vi "read tag bus from cvt.vi"(9 "Indices":i32[](array[numeric]), 10 "Data Type":T1, 11 "data table in":T2) -> (3 "data table out":T2)   [LabVIEW 2013, in "TEC runtime.lvclass"]
uses:
  TEC runtime.lvclass
  <vilib>/NI/Tag Bus/table/data table.ctl
  <vilib>/NI/Current Value Table/Type Defs/Data Types.ctl
  <vilib>/NI/Current Value Table/DataTypes/Double_Read Index Set.vi
  <vilib>/NI/Current Value Table/DataTypes/Array of String_Read Index Set.vi
  <vilib>/NI/Current Value Table/DataTypes/Array of Boolean_Read Index Set.vi
  <vilib>/NI/Current Value Table/DataTypes/Array of Single_Read Index Set.vi
  <vilib>/NI/Current Value Table/DataTypes/Array of Double_Read Index Set.vi
  <vilib>/NI/Current Value Table/DataTypes/Array of I8_Read Index Set.vi
  <vilib>/NI/Current Value Table/DataTypes/Array of I16_Read Index Set.vi
  <vilib>/NI/Current Value Table/DataTypes/Array of I32_Read Index Set.vi
  <vilib>/NI/Current Value Table/DataTypes/Array of I64_Read Index Set.vi
  <vilib>/NI/Current Value Table/DataTypes/Array of U64_Read Index Set.vi
  <vilib>/NI/Current Value Table/DataTypes/Array of U32_Read Index Set.vi
  <vilib>/NI/Current Value Table/DataTypes/Array of U16_Read Index Set.vi
  <vilib>/NI/Current Value Table/DataTypes/Array of U8_Read Index Set.vi
  <vilib>/NI/Current Value Table/DataTypes/Boolean_Read Index Set.vi
  <vilib>/NI/Current Value Table/DataTypes/String_Read Index Set.vi
  <vilib>/NI/Current Value Table/DataTypes/U8_Read Index Set.vi
  <vilib>/NI/Current Value Table/DataTypes/U16_Read Index Set.vi
  <vilib>/NI/Current Value Table/DataTypes/U32_Read Index Set.vi
  <vilib>/NI/Current Value Table/DataTypes/U64_Read Index Set.vi
  <vilib>/NI/Current Value Table/DataTypes/I8_Read Index Set.vi
  <vilib>/NI/Current Value Table/DataTypes/I16_Read Index Set.vi
  <vilib>/NI/Current Value Table/DataTypes/I32_Read Index Set.vi
  <vilib>/NI/Current Value Table/DataTypes/I64_Read Index Set.vi
  <vilib>/NI/Current Value Table/DataTypes/Single_Read Index Set.vi
  <vilib>/NI/Current Value Table/Memory Block.vi
  <vilib>/NI/Current Value Table/DataTypes/Double_Memory Block.vi
  <vilib>/NI/Current Value Table/DataTypes/Array of String_Memory Block.vi
  <vilib>/NI/Current Value Table/DataTypes/Array of Boolean_Memory Block.vi
  <vilib>/NI/Current Value Table/DataTypes/Array of Single_Memory Block.vi
  <vilib>/NI/Current Value Table/DataTypes/Array of Double_Memory Block.vi
  <vilib>/NI/Current Value Table/DataTypes/Array of I8_Memory Block.vi
  <vilib>/NI/Current Value Table/DataTypes/Array of I16_Memory Block.vi
  <vilib>/NI/Current Value Table/DataTypes/Array of I32_Memory Block.vi
  <vilib>/NI/Current Value Table/DataTypes/Array of I64_Memory Block.vi
  <vilib>/NI/Current Value Table/DataTypes/Array of U64_Memory Block.vi
  <vilib>/NI/Current Value Table/DataTypes/Array of U32_Memory Block.vi
  <vilib>/NI/Current Value Table/DataTypes/Array of U16_Memory Block.vi
  <vilib>/NI/Current Value Table/DataTypes/Array of U8_Memory Block.vi
  <vilib>/NI/Current Value Table/DataTypes/Boolean_Memory Block.vi
  <vilib>/NI/Current Value Table/DataTypes/String_Memory Block.vi
  <vilib>/NI/Current Value Table/DataTypes/U8_Memory Block.vi
  <vilib>/NI/Current Value Table/DataTypes/U16_Memory Block.vi
  <vilib>/NI/Current Value Table/DataTypes/U32_Memory Block.vi
  <vilib>/NI/Current Value Table/DataTypes/U64_Memory Block.vi
  <vilib>/NI/Current Value Table/DataTypes/I8_Memory Block.vi
  <vilib>/NI/Current Value Table/DataTypes/I16_Memory Block.vi
  <vilib>/NI/Current Value Table/DataTypes/I32_Memory Block.vi
  <vilib>/NI/Current Value Table/DataTypes/I64_Memory Block.vi
  <vilib>/NI/Current Value Table/DataTypes/Single_Memory Block.vi
  <vilib>/NI/Current Value Table/Current Value Table.lvlib
  <vilib>/NI/Tag Bus/table/data table.lvlib
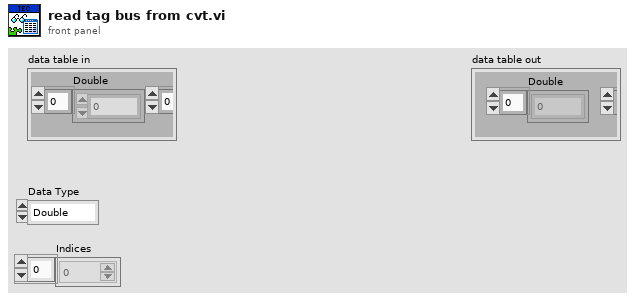
[diagram p1: front panel]
types:
  T1 = typedef "Current Value Table.lvlib/Data Types.ctl" = enum16{"Double", "Single", "I64", "I32", "I16", "I8", "U64", "U32", "U16", "U8", "String", "Boolean", "Array of U8", "Array of U16", "Array of U32", "Array of U64", "Array of I64", "Array of I32", "Array of I16", "Array of I8", "Array of Double", "Array of Single", "Array of Boolean", "Array of String"}
  T2 = typedef "tag bus.lvlib/data table.lvlib/data table.ctl" = cluster{"Double":dbl[], "Single":sgl[], "I64":i64[], "I32":i32[], "I16":i16[], "I8":i8[], "U64":u64[], "U32":u32[], "U16":u16[], "U8":u8[], "Boolean":bool[], "String":string[], "Array of Double":cluster{"DBL Array":dbl[]}[], "Array of Single":cluster{"SGL Array":sgl[]}[], "Array of I64":cluster{"I64 Array":i64[]}[], "Array of I32":cluster{"I32 Array":i32[]}[], "Array of I16":cluster{"I16 Array":i16[]}[], "Array of I8":cluster{"I8 Array":i8[]}[], "Array of U64":cluster{"U64 Array":u64[]}[], "Array of U32":cluster{"U32 Array":u32[]}[], "Array of U16":cluster{"U16 Array":u16[]}[], "Array of U8":cluster{"U8 Array":u8[]}[], "Array of Boolean":cluster{"Boolean Array":bool[]}[], "Array of String":cluster{"String Array":string[]}[]}
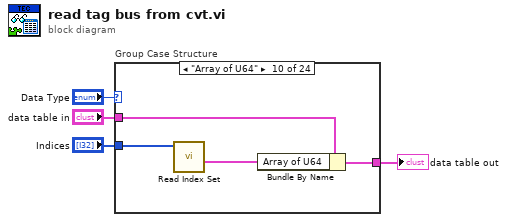
[diagram p0: block diagram]
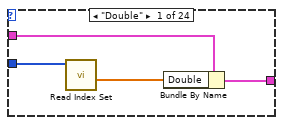
[diagram p2: hidden frame]
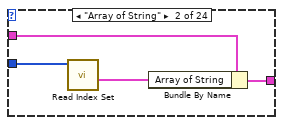
[diagram p3: hidden frame]
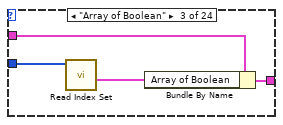
[diagram p4: hidden frame]
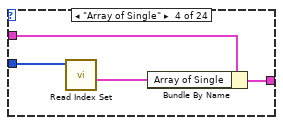
[diagram p5: hidden frame]
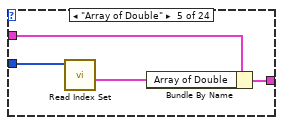
[diagram p6: hidden frame]
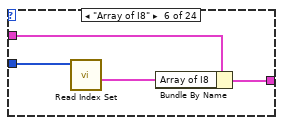
[diagram p7: hidden frame]
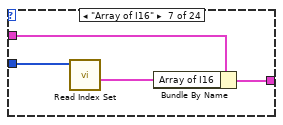
[diagram p8: hidden frame]
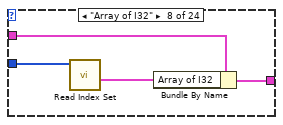
[diagram p9: hidden frame]
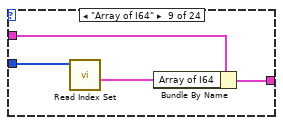
[diagram p10: hidden frame]
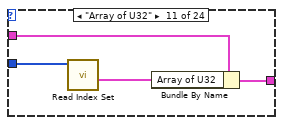
[diagram p11: hidden frame]
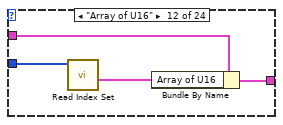
[diagram p12: hidden frame]
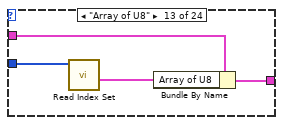
[diagram p13: hidden frame]
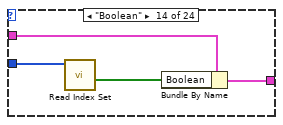
[diagram p14: hidden frame]
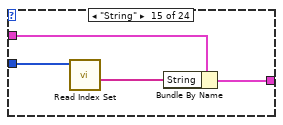
[diagram p15: hidden frame]
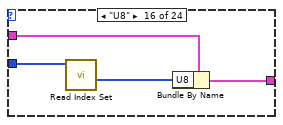
[diagram p16: hidden frame]
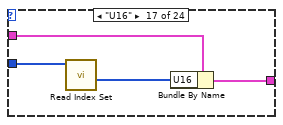
[diagram p17: hidden frame]
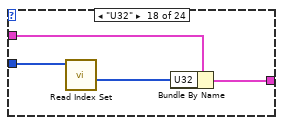
[diagram p18: hidden frame]
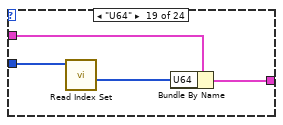
[diagram p19: hidden frame]
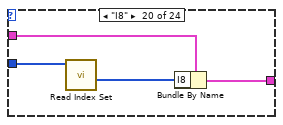
[diagram p20: hidden frame]
diagram:
  n1 = case "Group Case Structure" shown="\"Array of U64\"" "Data Type" {
    tunnel: "Indices" -> [w8 w12 w16 w20 w24 w28 w32 w36 w40 w44 w48 w52 w56 w60 w64 w68 w72 w76 w80 w84 w88 w92 w96 w100]
    tunnel: "data table in" -> [w7 w11 w15 w19 w23 w27 w31 w35 w39 w43 w47 w51 w55 w59 w63 w67 w71 w75 w79 w83 w87 w91 w95 w99]
    tunnel: [w6 w10 w14 w18 w22 w26 w30 w34 w38 w42 w46 w50 w54 w58 w62 w66 w70 w74 w78 w82 w86 w90 w94 w98] -> w3
    frame "Double" {
      n2 = call-poly <vilib>:"Read Index Set.vi"("Indices"=w8) -> ("Values"=w5:dbl[])  [unwired: 10 in]
      n3 = Bundle By Name(cluster=w7, "Double"=w5) -> (w6:T2)
    }
    frame "Array of String" {
      n4 = call-poly <vilib>:"Read Index Set.vi"("Indices"=w12) -> ("Values"=w9:cluster{"String Array":string[]}[])  [unwired: 10 in]
      n5 = Bundle By Name(cluster=w11, "Array of String"=w9) -> (w10:T2)
    }
    frame "Array of Boolean" {
      n6 = call-poly <vilib>:"Read Index Set.vi"("Indices"=w16) -> ("Values"=w13:cluster{"Boolean Array":bool[]}[])  [unwired: 10 in]
      n7 = Bundle By Name(cluster=w15, "Array of Boolean"=w13) -> (w14:T2)
    }
    frame "Array of Single" {
      n8 = call-poly <vilib>:"Read Index Set.vi"("Indices"=w20) -> ("Values"=w17:cluster{"SGL Array":sgl[]}[])  [unwired: 10 in]
      n9 = Bundle By Name(cluster=w19, "Array of Single"=w17) -> (w18:T2)
    }
    frame "Array of Double" {
      n10 = call-poly <vilib>:"Read Index Set.vi"("Indices"=w24) -> ("Values"=w21:cluster{"DBL Array":dbl[]}[])  [unwired: 10 in]
      n11 = Bundle By Name(cluster=w23, "Array of Double"=w21) -> (w22:T2)
    }
    frame "Array of I8" {
      n12 = call-poly <vilib>:"Read Index Set.vi"("Indices"=w28) -> ("Values"=w25:cluster{"I8 Array":i8[]}[])  [unwired: 10 in]
      n13 = Bundle By Name(cluster=w27, "Array of I8"=w25) -> (w26:T2)
    }
    frame "Array of I16" {
      n14 = call-poly <vilib>:"Read Index Set.vi"("Indices"=w32) -> ("Values"=w29:cluster{"I16 Array":i16[]}[])  [unwired: 10 in]
      n15 = Bundle By Name(cluster=w31, "Array of I16"=w29) -> (w30:T2)
    }
    frame "Array of I32" {
      n16 = call-poly <vilib>:"Read Index Set.vi"("Indices"=w36) -> ("Values"=w33:cluster{"I32 Array":i32[]}[])  [unwired: 10 in]
      n17 = Bundle By Name(cluster=w35, "Array of I32"=w33) -> (w34:T2)
    }
    frame "Array of I64" {
      n18 = call-poly <vilib>:"Read Index Set.vi"("Indices"=w40) -> ("Values"=w37:cluster{"I64 Array":i64[]}[])  [unwired: 10 in]
      n19 = Bundle By Name(cluster=w39, "Array of I64"=w37) -> (w38:T2)
    }
    frame "Array of U64" {
      n20 = call-poly <vilib>:"Read Index Set.vi"("Indices"=w44) -> ("Values"=w41:cluster{"U64 Array":u64[]}[])  [unwired: 10 in]
      n21 = Bundle By Name(cluster=w43, "Array of U64"=w41) -> (w42:T2)
    }
    frame "Array of U32" {
      n22 = call-poly <vilib>:"Read Index Set.vi"("Indices"=w48) -> ("Values"=w45:cluster{"U32 Array":u32[]}[])  [unwired: 10 in]
      n23 = Bundle By Name(cluster=w47, "Array of U32"=w45) -> (w46:T2)
    }
    frame "Array of U16" {
      n24 = call-poly <vilib>:"Read Index Set.vi"("Indices"=w52) -> ("Values"=w49:cluster{"U16 Array":u16[]}[])  [unwired: 10 in]
      n25 = Bundle By Name(cluster=w51, "Array of U16"=w49) -> (w50:T2)
    }
    frame "Array of U8" {
      n26 = call-poly <vilib>:"Read Index Set.vi"("Indices"=w56) -> ("Values"=w53:cluster{"U8 Array":u8[]}[])  [unwired: 10 in]
      n27 = Bundle By Name(cluster=w55, "Array of U8"=w53) -> (w54:T2)
    }
    frame "Boolean" {
      n28 = call-poly <vilib>:"Read Index Set.vi"("Indices"=w60) -> ("Values"=w57:bool[])  [unwired: 10 in]
      n29 = Bundle By Name(cluster=w59, "Boolean"=w57) -> (w58:T2)
    }
    frame "String" {
      n30 = call-poly <vilib>:"Read Index Set.vi"("Indices"=w64) -> ("Values"=w61:string[])  [unwired: 10 in]
      n31 = Bundle By Name(cluster=w63, "String"=w61) -> (w62:T2)
    }
    frame "U8" {
      n32 = call-poly <vilib>:"Read Index Set.vi"("Indices"=w68) -> ("Values"=w65:u8[])  [unwired: 10 in]
      n33 = Bundle By Name(cluster=w67, "U8"=w65) -> (w66:T2)
    }
    frame "U16" {
      n34 = call-poly <vilib>:"Read Index Set.vi"("Indices"=w72) -> ("Values"=w69:u16[])  [unwired: 10 in]
      n35 = Bundle By Name(cluster=w71, "U16"=w69) -> (w70:T2)
    }
    frame "U32" {
      n36 = call-poly <vilib>:"Read Index Set.vi"("Indices"=w76) -> ("Values"=w73:u32[])  [unwired: 10 in]
      n37 = Bundle By Name(cluster=w75, "U32"=w73) -> (w74:T2)
    }
    frame "U64" {
      n38 = call-poly <vilib>:"Read Index Set.vi"("Indices"=w80) -> ("Values"=w77:u64[])  [unwired: 10 in]
      n39 = Bundle By Name(cluster=w79, "U64"=w77) -> (w78:T2)
    }
    frame "I8" {
      n40 = call-poly <vilib>:"Read Index Set.vi"("Indices"=w84) -> ("Values"=w81:i8[])  [unwired: 10 in]
      n41 = Bundle By Name(cluster=w83, "I8"=w81) -> (w82:T2)
    }
    frame "I16" {
      n42 = call-poly <vilib>:"Read Index Set.vi"("Indices"=w88) -> ("Values"=w85:i16[])  [unwired: 10 in]
      n43 = Bundle By Name(cluster=w87, "I16"=w85) -> (w86:T2)
    }
    frame "I32" {
      n44 = call-poly <vilib>:"Read Index Set.vi"("Indices"=w92) -> ("Values"=w89:i32[])  [unwired: 10 in]
      n45 = Bundle By Name(cluster=w91, "I32"=w89) -> (w90:T2)
    }
    frame "I64" {
      n46 = call-poly <vilib>:"Read Index Set.vi"("Indices"=w96) -> ("Values"=w93:i64[])  [unwired: 10 in]
      n47 = Bundle By Name(cluster=w95, "I64"=w93) -> (w94:T2)
    }
    frame "Single" {
      n48 = call-poly <vilib>:"Read Index Set.vi"("Indices"=w100) -> ("Values"=w97:sgl[])  [unwired: 10 in]
      n49 = Bundle By Name(cluster=w99, "Single"=w97) -> (w98:T2)
    }
  }
  "data table out" <- w3
